vi "Ask_561_on.vi"(8 "error in":errorcluster, 11 "VISA resource name":refnum<visa-resource-name>) -> (0 "error out":errorcluster, 2 "561 On":bool, 3 "VISA resource name out":refnum<visa-resource-name>)   [LabVIEW 2015]
panel:
  out "Serial Settings:Number of Bytes at Serial Port":u32
  out "read buffer":string
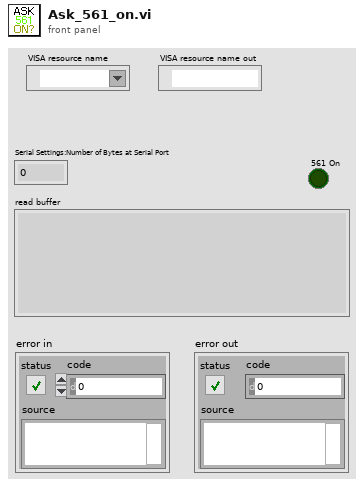
[diagram p1: front panel]
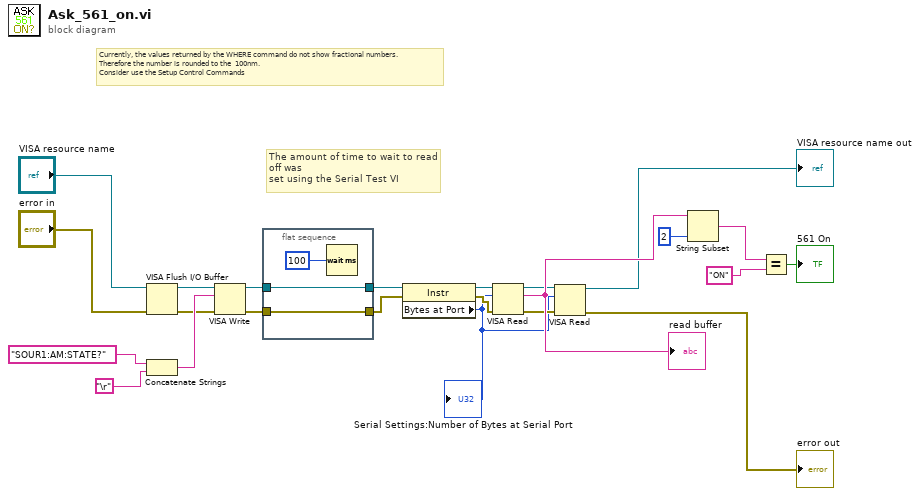
[diagram p0: block diagram]
diagram:
  # "Currently, the values returned by the WHERE command do not show fractional numbers.\nTherefore the number is rounded to the  100nm. \nConsider use the Setup Control Commands"
  # "The amount of time to wait to read off was \nset using the Serial Test VI"
  n1 = VISA Flush I/O Buffer(VISA resource name="VISA resource name", error in (no error)="error in") -> (VISA resource name out=w4:refnum<visa-resource-name>, error out=w1:errorcluster)  [unwired: 1 in]
  n2 = Concatenate Strings("SOUR1:AM:STATE?" ("string"), "\r") -> (w17:string)
  n3 = VISA Write(VISA resource name=w4, write buffer=w17, error in (no error)=w1) -> (VISA resource name out=w21:refnum<visa-resource-name>, error out=w19:errorcluster)  [unwired: 1 out]
  n4 = flat-sequence {
    tunnel: [w26] -> w22
    tunnel: w21 -> [w26]
    tunnel: [w24] -> w20
    tunnel: w19 -> [w24]
    frame #0 {
      n5 = Wait (ms)(milliseconds to wait=u32 100) -> ()  [unwired: 1 out]
    }
  }
  n6 = property class="Instr"(reference=w22, error in=w20) -> (reference out=w23:refnum<visa-resource-name>, error out=w18:errorcluster, "Bytes at Port"=w7:u32)
  "Serial Settings:Number of Bytes at Serial Port" <- w7
  n7 = VISA Read(VISA resource name=w23, byte count=w7, error in (no error)=w18) -> (VISA resource name out=w8:refnum<visa-resource-name>, read buffer=w12:string, error out=w9:errorcluster)  [unwired: 1 out]
  "read buffer" <- w12
  n8 = VISA Read(VISA resource name=w8, byte count=w7, error in (no error)=w9) -> (VISA resource name out=→"VISA resource name out":refnum<visa-resource-name>, error out=→"error out":errorcluster)  [unwired: 2 out]
  n9 = String Subset(string=w12, length (rest)=2 ("length (rest)")) -> (substring=w11:string)  [unwired: 1 in]
  n10 = Equal?(x=w11, y="ON" ("regular expression")) -> (x = y?=→"561 On":bool)
